vi "Wave2D_Cal Uk_ADI V.vi"(10 "time step":i32, 11 "Wave2D Data In":T1={"PDE"={"k"=0.0, "a"=0.0, "F(t, x, y)"=[]}, "Domain"={"t"={"initial t"=0.0, "final t"=0.0, "# of t-points"=0}, "x"={"start x"=0.0, "end x"=0.0, "# of x-points"=0}, "y"={"start y"=0.0, "end y"=0.0, "# of y-points"=11}, "delta"={"delta t"=0.0, "delta x"=0.0, "delta y"=0.0}}, "BC"={"Start X"={"type"=0, "Value"=[]}, "End X"={"type"=0, "Value"=[]}, "Start Y"={"type"=0, "Value"=[]}, "End Y"={"type"=0, "Value"=[]}}, "Corner"={"Start X & Start Y"=[], "Start X & End Y"=[], "End X & Start Y"=[], "End X & End Y"=[]}, "IC"={"Value"=[], "Derivative"=[]}, "P"={"Sub Diag"=[], "Diag"=[], "Super Diag"=[], "P"=[]}, "LU of P"={"L"=[], "U"={"Diag"=[], "Super Diag"=[], "2nd Super Diag"=[]}, "Pivot"=[]}, "Q"={"Sub Diag"=[], "Diag"=[], "Super Diag"=[], "Q"=[]}, "LU of Q"={"L"=[], "U"={"Diag"=[], "Super Diag"=[], "2nd Super Diag"=[]}, "Pivot"=[]}, "State"={"U"=[], "Old U"=[], "V&W"=[], "x start index"=0, "x length"=0, "y start index"=0, "y length"=0}} {"BC"."End Y"."type" items=["Dirichlet", "Neumann"]; "BC"."Start Y"."type" items=["Dirichlet", "Neumann"]; "BC"."End X"."type" items=["Dirichlet", "Neumann"]; "BC"."Start X"."type" items=["Dirichlet", "Neumann"]}) -> (3 "Wave2D Data Out":T1={"PDE"={"k"=0.0, "a"=0.0, "F(t, x, y)"=[]}, "Domain"={"t"={"initial t"=0.0, "final t"=0.0, "# of t-points"=0}, "x"={"start x"=0.0, "end x"=0.0, "# of x-points"=0}, "y"={"start y"=0.0, "end y"=0.0, "# of y-points"=11}, "delta"={"delta t"=0.0, "delta x"=0.0, "delta y"=0.0}}, "BC"={"Start X"={"type"=0, "Value"=[]}, "End X"={"type"=0, "Value"=[]}, "Start Y"={"type"=0, "Value"=[]}, "End Y"={"type"=0, "Value"=[]}}, "Corner"={"Start X & Start Y"=[], "Start X & End Y"=[], "End X & Start Y"=[], "End X & End Y"=[]}, "IC"={"Value"=[], "Derivative"=[]}, "P"={"Sub Diag"=[], "Diag"=[], "Super Diag"=[], "P"=[]}, "LU of P"={"L"=[], "U"={"Diag"=[], "Super Diag"=[], "2nd Super Diag"=[]}, "Pivot"=[]}, "Q"={"Sub Diag"=[], "Diag"=[], "Super Diag"=[], "Q"=[]}, "LU of Q"={"L"=[], "U"={"Diag"=[], "Super Diag"=[], "2nd Super Diag"=[]}, "Pivot"=[]}, "State"={"U"=[], "Old U"=[], "V&W"=[], "x start index"=0, "x length"=0, "y start index"=0, "y length"=0}} {"BC"."End Y"."type" items=["Dirichlet", "Neumann"]; "BC"."Start Y"."type" items=["Dirichlet", "Neumann"]; "BC"."End X"."type" items=["Dirichlet", "Neumann"]; "BC"."Start X"."type" items=["Dirichlet", "Neumann"]})   [LabVIEW 2020, in "NI_PDE.lvlib"]
uses:
  <vilib>/gmath/NI_PDE.lvlib
  <vilib>/gmath/pde.llb/Wave2D/Wave2D_Data.ctl
  <vilib>/gmath/pde.llb/Common/PDE_BC Type.ctl
  <vilib>/Analysis/Matrix/Datatypes/RealMatrix.ctl
  <vilib>/Analysis/Matrix/NI_Matrix.lvlib
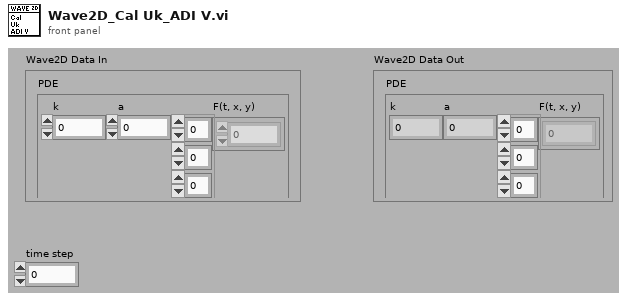
[diagram p1: front panel]
types:
  T1 = typedef "NI_PDE.lvlib/Wave2D_Data.ctl" = cluster{"PDE":cluster{"k":dbl, "a":dbl, "F(t, x, y)":dbl[][][]}, "Domain":cluster{"t":cluster{"initial t":dbl, "final t":dbl, "# of t-points":i32}, "x":cluster{"start x":dbl, "end x":dbl, "# of x-points":i32}, "y":cluster{"start y":dbl, "end y":dbl, "# of y-points":i32}, "delta":cluster{"delta t":dbl, "delta x":dbl, "delta y":dbl}}, "BC":cluster{"Start X":cluster{"type":T2, "Value":dbl[][]}, "End X":cluster{"type":T2, "Value":dbl[][]}, "Start Y":cluster{"type":T2, "Value":dbl[][]}, "End Y":cluster{"type":T2, "Value":dbl[][]}}, "Corner":cluster{"Start X & Start Y":dbl[], "Start X & End Y":dbl[], "End X & Start Y":dbl[], "End X & End Y":dbl[]}, "IC":cluster{"Value":dbl[][], "Derivative":dbl[][]}, "P":cluster{"Sub Diag":dbl[], "Diag":dbl[], "Super Diag":dbl[], "P":T3}, "LU of P":cluster{"L":dbl[], "U":cluster{"Diag":dbl[], "Super Diag":dbl[], "2nd Super Diag":dbl[]}, "Pivot":i32[]}, "Q":cluster{"Sub Diag":dbl[], "Diag":dbl[], "Super Diag":dbl[], "Q":T3}, "LU of Q":cluster{"L":dbl[], "U":cluster{"Diag":dbl[], "Super Diag":dbl[], "2nd Super Diag":dbl[]}, "Pivot":i32[]}, "State":cluster{"U":dbl[][], "Old U":dbl[][], "V&W":dbl[][], "x start index":i32, "x length":i32, "y start index":i32, "y length":i32}}
  T2 = typedef "NI_PDE.lvlib/PDE_BC Type.ctl" = i32
  T3 = typedef "NI_Matrix.lvlib/RealMatrix.ctl" = dbl[][]
  T4 = cluster{"L":dbl[], "U":cluster{"Diag":dbl[], "Super Diag":dbl[], "2nd Super Diag":dbl[]}, "Pivot":i32[]}
  T5 = cluster{"Start X & Start Y":dbl[], "Start X & End Y":dbl[], "End X & Start Y":dbl[], "End X & End Y":dbl[]}
  T6 = cluster{"Sub Diag":dbl[], "Diag":dbl[], "Super Diag":dbl[], "P":T3}
  T7 = cluster{"Sub Diag":dbl[], "Diag":dbl[], "Super Diag":dbl[], "Q":T3}
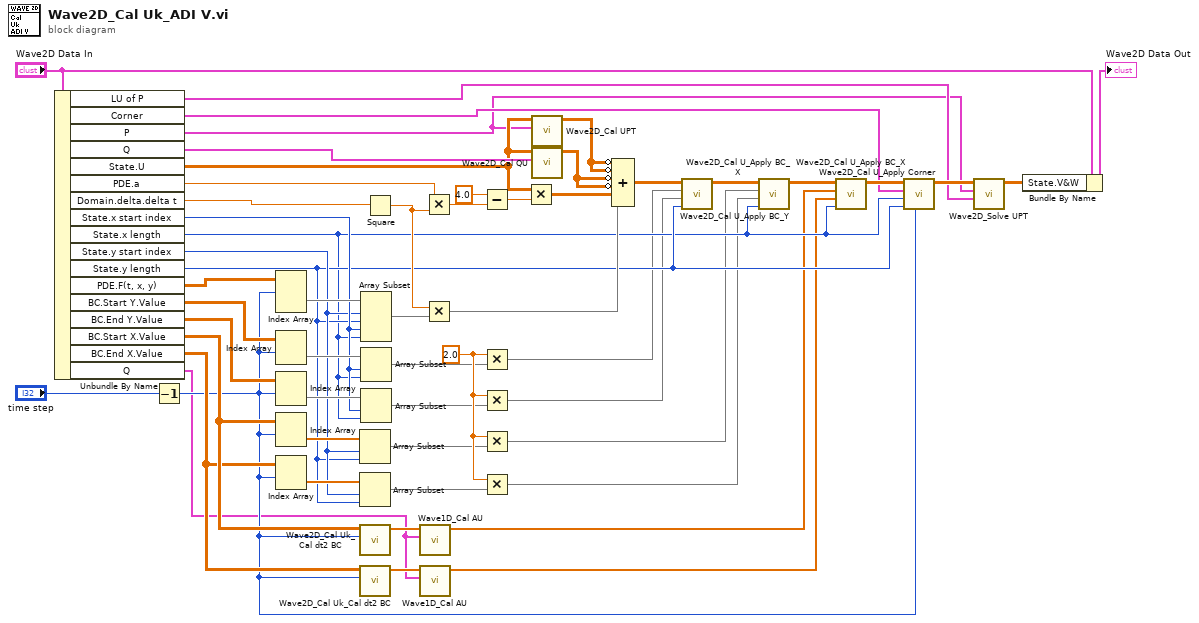
[diagram p0: block diagram]
diagram:
  w11 = 2.0 ("x")
  n1 = Unbundle By Name("Wave2D Data In") -> ("LU of P"=w20:T4, "Corner"=w24:T5, "P"=w17:T6, "Q"=w19:T7, "State.U"=w18:dbl[][], "PDE.a"=w50:dbl, "Domain.delta.delta t"=w47:dbl, "State.x start index"=w33:i32, "State.x length"=w12:i32, "State.y start index"=w30:i32, "State.y length"=w13:i32, "PDE.F(t, x, y)"=w46:dbl[][][], "BC.Start Y.Value"=w37:dbl[][], "BC.End Y.Value"=w35:dbl[][], "BC.Start X.Value"=w29:dbl[][], "BC.End X.Value"=w27:dbl[][], "Q"=w14:T7)
  n2 = Decrement(x="time step") -> (x-1=w23:i32)
  n3 = Index Array(array=w46, index (dim 0)=w23) -> (element=w45:dbl[][])  [unwired: 2 in]
  n4 = Index Array(array=w37, index (row)=w23) -> (element=w36:dbl[])  [unwired: 1 in]
  n5 = Index Array(array=w35, index (row)=w23) -> (element=w34:dbl[])  [unwired: 1 in]
  n6 = Index Array(array=w29, index (row)=w23) -> (element=w32:dbl[])  [unwired: 1 in]
  n7 = Index Array(array=w27, index (row)=w23) -> (element=w31:dbl[])  [unwired: 1 in]
  n8 = Array Subset(array=w32, index=w30, length=w13) -> (w6:dbl[])
  n9 = Array Subset(array=w31, index=w30, length=w13) -> (w4:dbl[])
  n10 = call <vilib>:"Wave2D_Cal Uk_Cal dt2 BC.vi"("time step"=w23, "BC Value"=w29) -> ("dt2 BC"=w16:dbl[])  [unwired: 9 out]
  n11 = call <vilib>:"Wave2D_Cal Uk_Cal dt2 BC.vi"("time step"=w23, "BC Value"=w27) -> ("dt2 BC"=w15:dbl[])  [unwired: 9 out]
  n12 = Array Subset(array=w45, index (row)=w30, length (row)=w13, index (col)=w33, length (col)=w12) -> (w44:dbl[][])
  n13 = Array Subset(array=w36, index=w33, length=w12) -> (w10:dbl[])
  n14 = Array Subset(array=w34, index=w33, length=w12) -> (w8:dbl[])
  n15 = Square(x=w47) -> (x^2=w42:dbl)
  n16 = call <vilib>:"Wave1D_Cal AU.vi"("A"=w14, "U"=w16) -> ("AU"=w2:dbl[])  [unwired: 9 out]
  n17 = call <vilib>:"Wave1D_Cal AU.vi"("A"=w14, "U"=w15) -> ("AU"=w1:dbl[])  [unwired: 9 out]
  n18 = Multiply(x=w50, y=w42) -> (x*y=w52:dbl)
  n19 = Multiply(x=w42, y=w44) -> (x*y=w43:dbl[][])
  n20 = Subtract(x=4.0, y=w52) -> (x-y=w49:dbl)
  n21 = Multiply(x=w11, y=w10) -> (x*y=w9:dbl[])
  n22 = Multiply(x=w11, y=w8) -> (x*y=w7:dbl[])
  n23 = Multiply(x=w11, y=w6) -> (x*y=w5:dbl[])
  n24 = Multiply(x=w11, y=w4) -> (x*y=w3:dbl[])
  n25 = Multiply(x=w18, y=w49) -> (x*y=w48:dbl[][])
  n26 = call <vilib>:"Wave2D_Cal UPT.vi"("P"=w17, "U"=w18) -> ("UPT"=w40:dbl[][])  [unwired: 9 out]
  n27 = call <vilib>:"Wave2D_Cal QU.vi"("Q"=w19, "U"=w18) -> ("QU"=w41:dbl[][])  [unwired: 9 out]
  n28 = Compound Arithmetic op=ADD(invert w40, invert w40, invert w41, invert w41, w48, w43) -> (w38:dbl[][])
  n29 = call <vilib>:"Wave2D_Cal U_Apply BC_Y.vi"("y length"=w13, "End Y Value"=w7, "Start Y Value"=w9, "U In"=w38) -> ("U Out"=w39:dbl[][])  [unwired: 2 in, 5 out]
  n30 = call <vilib>:"Wave2D_Cal U_Apply BC_X.vi"("x length"=w12, "End X Value"=w3, "Start X Value"=w5, "U In"=w39) -> ("U Out"=w26:dbl[][])  [unwired: 2 in, 5 out]
  n31 = call <vilib>:"Wave2D_Cal U_Apply BC_X.vi"("x length"=w12, "End X Value"=w1, "Start X Value"=w2, "U In"=w26) -> ("U Out"=w25:dbl[][])  [unwired: 2 in, 5 out]
  n32 = call <vilib>:"Wave2D_Cal U_Apply Corner.vi"("time step"=w23, "y length"=w13, "x length"=w12, "Corner"=w24, "U In"=w25) -> ("U Out"=w21:dbl[][])  [unwired: 6 out]
  n33 = call <vilib>:"Wave2D_Solve UPT.vi"("LU of P"=w20, "P"=w17, "U"=w21) -> ("U/PT"=w22:dbl[][])  [unwired: 8 out]
  n34 = Bundle By Name(cluster="Wave2D Data In", "State.V&W"=w22) -> (→"Wave2D Data Out":T1)
